vi "TestExec.Config, Get Station SW Module Info - Old.vi"(7 "Error if EXE does not exist":bool, 8 "Error if File Doesn't Exist":bool, 9 "Create File if Doesn't Exist":bool, 11 "Path":path=path "C:/MTE/Test Executive/Config") -> (0 "error out":errorcluster, 1 "Station IP Port":i32, 2 "Station Name":string, 3 "Sta Exe Path":path)   [LabVIEW 2018]
uses:
  <vilib>/Utility/config.llb/Read Key (String).vi
  <vilib>/Utility/config.llb/Read Key (I32).vi
  <vilib>/Utility/config.llb/Read Key (Path).vi
  <vilib>/Utility/config.llb/NI_LVConfig.lvlib
  <vilib>/KATE/Files/File Utils.lvlib
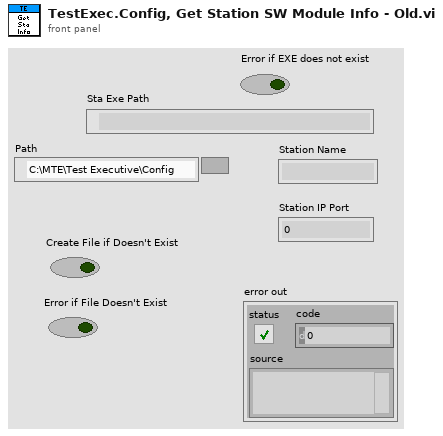
[diagram p1: front panel]
types:
  T1 = typedef "NI_LVConfig.lvlib/Config Data RefNum.ctl" = refnum<k1>
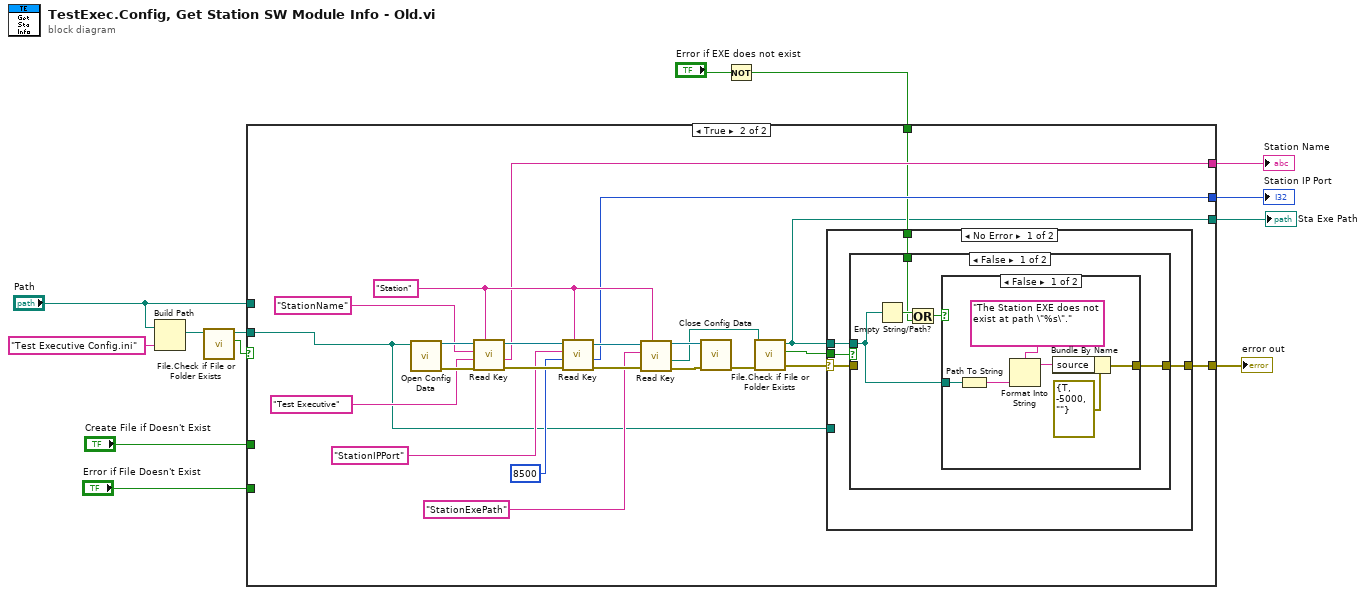
[diagram p0: block diagram]
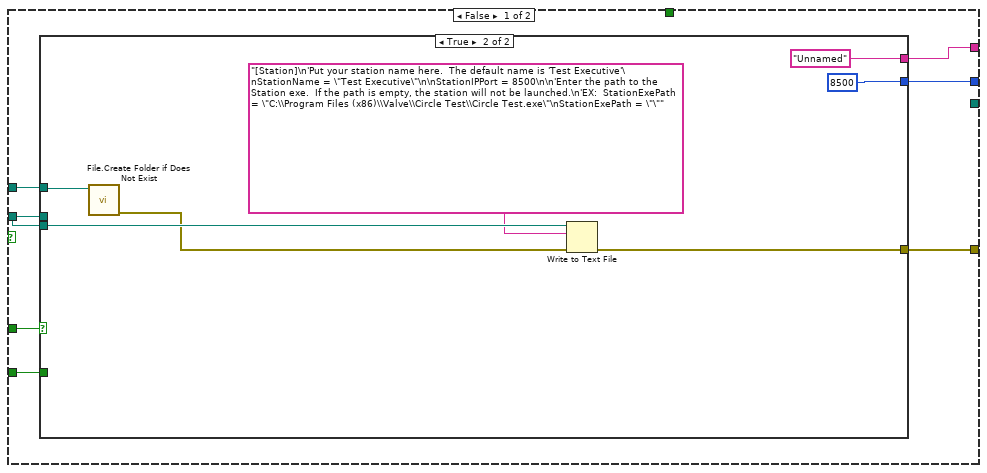
[diagram p2: hidden frame]
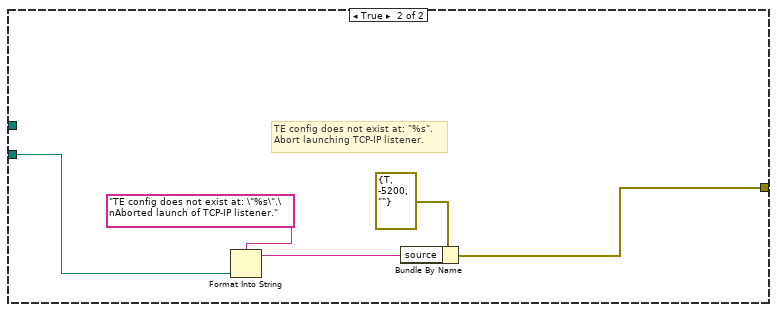
[diagram p4: hidden frame]
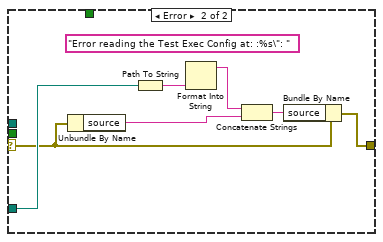
[diagram p7: hidden frame]
diagram:
  n1 = Build Path(base path="Path", name or relative path="Test Executive Config.ini") -> (appended path=w11:path)
  n2 = call <vilib>:"File.Check if File or Folder Exists.vi"("Path"=w11) -> ("Exists"=w9:bool, "Dup Path"=w10:path)  [unwired: 6 in, 3 out]
  n3 = Not(x="Error if EXE does not exist") -> (.not. x?=w2:bool)
  n4 = case shown="True" w9 {
    tunnel: [w20 w57] -> w13
    tunnel: w10 -> [w15 w41]
    tunnel: "Create File if Doesn't Exist" -> [w19 _]
    tunnel: [w17 w40] -> w7
    tunnel: [w18 w39] -> w6
    tunnel: "Error if File Doesn't Exist" -> [w16 _]
    tunnel: "Path" -> [w14 _]
    tunnel: w2 -> [_ w38]
    tunnel: [_ w37] -> w1
    frame False {
      n5 = case shown="True" w19 {
        tunnel: w15 -> [_ w36]
        tunnel: [w22 w34] -> w20
        tunnel: [_ 8500] -> w18
        tunnel: [_ "Unnamed"] -> w17
        tunnel: w16 -> [w24 _]
        tunnel: w15 -> [w23 _]
        tunnel: w14 -> [w21 w31]
        frame False {
          n6 = case shown="False" w24 {
            tunnel: w23 -> [_ w28]
            tunnel: [_ w25] -> w22
            tunnel: w21 -> [_ _]
            frame False {
            }
            frame True {
              # "TE config does not exist at: \"%s\".\nAbort launching TCP-IP listener."
              n7 = Format Into String(format string="TE config does not exist at: \"%s\".\nAborted launch of TCP-IP listener." ("source"), w28) -> (resulting string=w26:string)  [unwired: 2 in, 1 out]
              n8 = Bundle By Name(cluster=errorcluster {"status"=TRUE, "code"=-5200, "source"=""} ("error constant"), "source"=w26) -> (w25:errorcluster)
            }
          }
        }
        frame True {
          n9 = call <vilib>:"File.Create Folder if Does Not Exist.vi"("Path"=w31) -> ("error out"=w30:errorcluster)  [unwired: 8 in, 2 out]
          n10 = Write to Text File(file (use dialog)=w36, text="[Station]\n'Put your station name here.  The default name is 'Test Executive'\nStationName = \"Test Executive\"\n\nStationIPPort = 8500\n\n'Enter the path to the Station exe.  If the path is empty, the station will not be launched.\n'EX:  StationExePath = \"C:\\Program Files (x86)\\Valve\\Circle Test\\Circle Test.exe\"\nStationExePath = \"\"", error in=w30) -> (error out=w34:errorcluster)  [unwired: 1 in, 2 out]
        }
      }
    }
    frame True {
      w47 = "Station" ("section")
      n11 = call <vilib>:"Open Config Data.vi"("configuration file path"=w41) -> ("error out"=w55:errorcluster, "refnum"=w56:T1)  [unwired: 8 in, 1 out]
      n12 = call-poly <vilib>:"Read Key.vi"("section"=w47, "error in (no error)"=w55, "default value"="Test Executive" ("section"), "key"="StationName" ("section"), "refnum"=w56) -> ("error out"=w54:errorcluster, "value"=w40:string, "refnum out"=w53:T1)  [unwired: 3 in, 1 out]
      n13 = call-poly <vilib>:"Read Key.vi"("section"=w47, "error in (no error)"=w54, "default value"=8500, "key"="StationIPPort", "refnum"=w53) -> ("error out"=w50:errorcluster, "value"=w39:i32, "refnum out"=w51:T1)  [unwired: 3 in, 1 out]
      n14 = call-poly <vilib>:"Read Key.vi"("section"=w47, "error in (no error)"=w50, "key"="StationExePath", "refnum"=w51) -> ("error out"=w49:errorcluster, "value"=w43:path, "refnum out"=w48:T1)  [unwired: 4 in, 1 out]
      n15 = call <vilib>:"Close Config Data.vi"("error in (no error)"=w49, "refnum"=w48) -> ("error out"=w60:errorcluster)  [unwired: 8 in, 1 out]
      n16 = call <vilib>:"File.Check if File or Folder Exists.vi"("error in"=w60, "Path"=w43) -> ("error out"=w59:errorcluster, "Exists"=w58:bool, "Dup Path"=w37:path)  [unwired: 5 in, 2 out]
      n17 = case shown="No Error" w59 {
        selector: w59 -> [w63 w79]
        tunnel: w58 -> [w65 _]
        tunnel: w37 -> [w64 _]
        tunnel: [w62 w78] -> w57
        tunnel: w41 -> [_ w83]
        tunnel: w38 -> [w61 _]
        frame No Error {
          n18 = case shown="False" w65 {
            tunnel: w64 -> [w69 _]
            tunnel: w63 -> [_ w77]
            tunnel: [w70 w77] -> w62
            tunnel: w61 -> [w66 _]
            frame False {
              n19 = Empty String/Path?(string/path=w69) -> (empty?=w68:bool)
              n20 = Or(x=w68, y=w66) -> (x .or. y?=w67:bool)
              n21 = case shown="False" w67 {
                tunnel: [w72 _] -> w70
                tunnel: w69 -> [w71 _]
                frame False {
                  n22 = Path To String(path=w71) -> (string=w76:string)
                  n23 = Format Into String(format string="The Station EXE does not exist at path \"%s\".", w76) -> (resulting string=w74:string)  [unwired: 2 in, 1 out]
                  n24 = Bundle By Name(cluster=errorcluster {"status"=TRUE, "code"=-5000, "source"=""} ("error constant"), "source"=w74) -> (w72:errorcluster)
                }
                frame True {
                }
              }
            }
            frame True {
            }
          }
        }
        frame Error {
          (unwired) "Error reading the Test Exec Config at: :%s\": "
          n25 = Unbundle By Name(w79) -> ("source"=w81:string)
          n26 = Path To String(path=w83) -> (string=w84:string)
          n27 = Format Into String(w84) -> (resulting string=w82:string)  [unwired: 3 in, 1 out]
          n28 = Concatenate Strings(w82, w81) -> (w80:string)
          n29 = Bundle By Name(cluster=w79, "source"=w80) -> (w78:errorcluster)
        }
      }
    }
  }
  "error out" <- w13
  "Station Name" <- w7
  "Station IP Port" <- w6
  "Sta Exe Path" <- w1
